vi "DC Offset.vi"() -> ()   [LabVIEW 2018]
uses:
  <vilib>/Analysis/baseanly.llb/Mean (DBL).vi
  <vilib>/express/express shared/transition.llb/Dynamic To Waveform Array.vi
  <vilib>/express/express signal manip/GetorSetDDTAttributes/Set DDT Attributes/SetT0.vi
  <vilib>/express/express shared/transition.llb/Waveform Array To Dynamic.vi
  <vilib>/express/express signal manip/GetorSetDDTAttributes/Set DDT Attributes/Set DDT Properties.xnode
  <vilib>/Analysis/NI_AALBase.lvlib
panel:
  in  "Filename":path=path "C:/Users/physics-svc-fulda/Desktop/LabVIEW Data/DC OFFset.lvm"
  out "Waveform Graph":dynamicdata(graph)
  out "Saving Data":bool
  in  "Enable":bool=TRUE
  out "DC D":dbl format="%0.6f"
  out "DC C":dbl format="%0.6f"
  out "DC B":dbl format="%0.6f"
  out "DC A":dbl format="%0.6f"
  in  "timeout (s)":dbl=10.0 format="%0.2f"
  in  "rate":dbl=1000.0
  in  "# of samples":i32=100
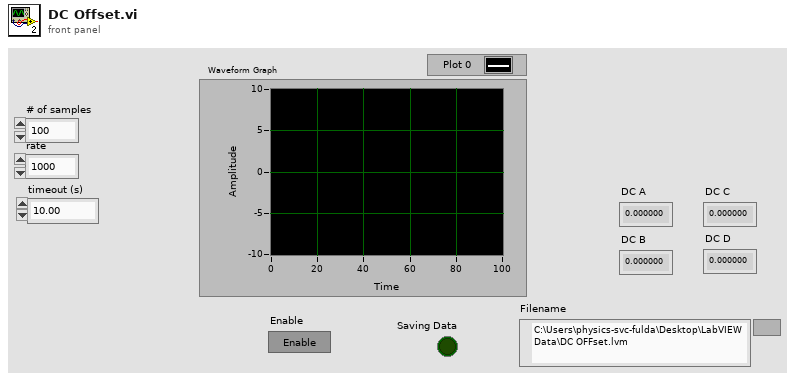
[diagram p1: front panel]
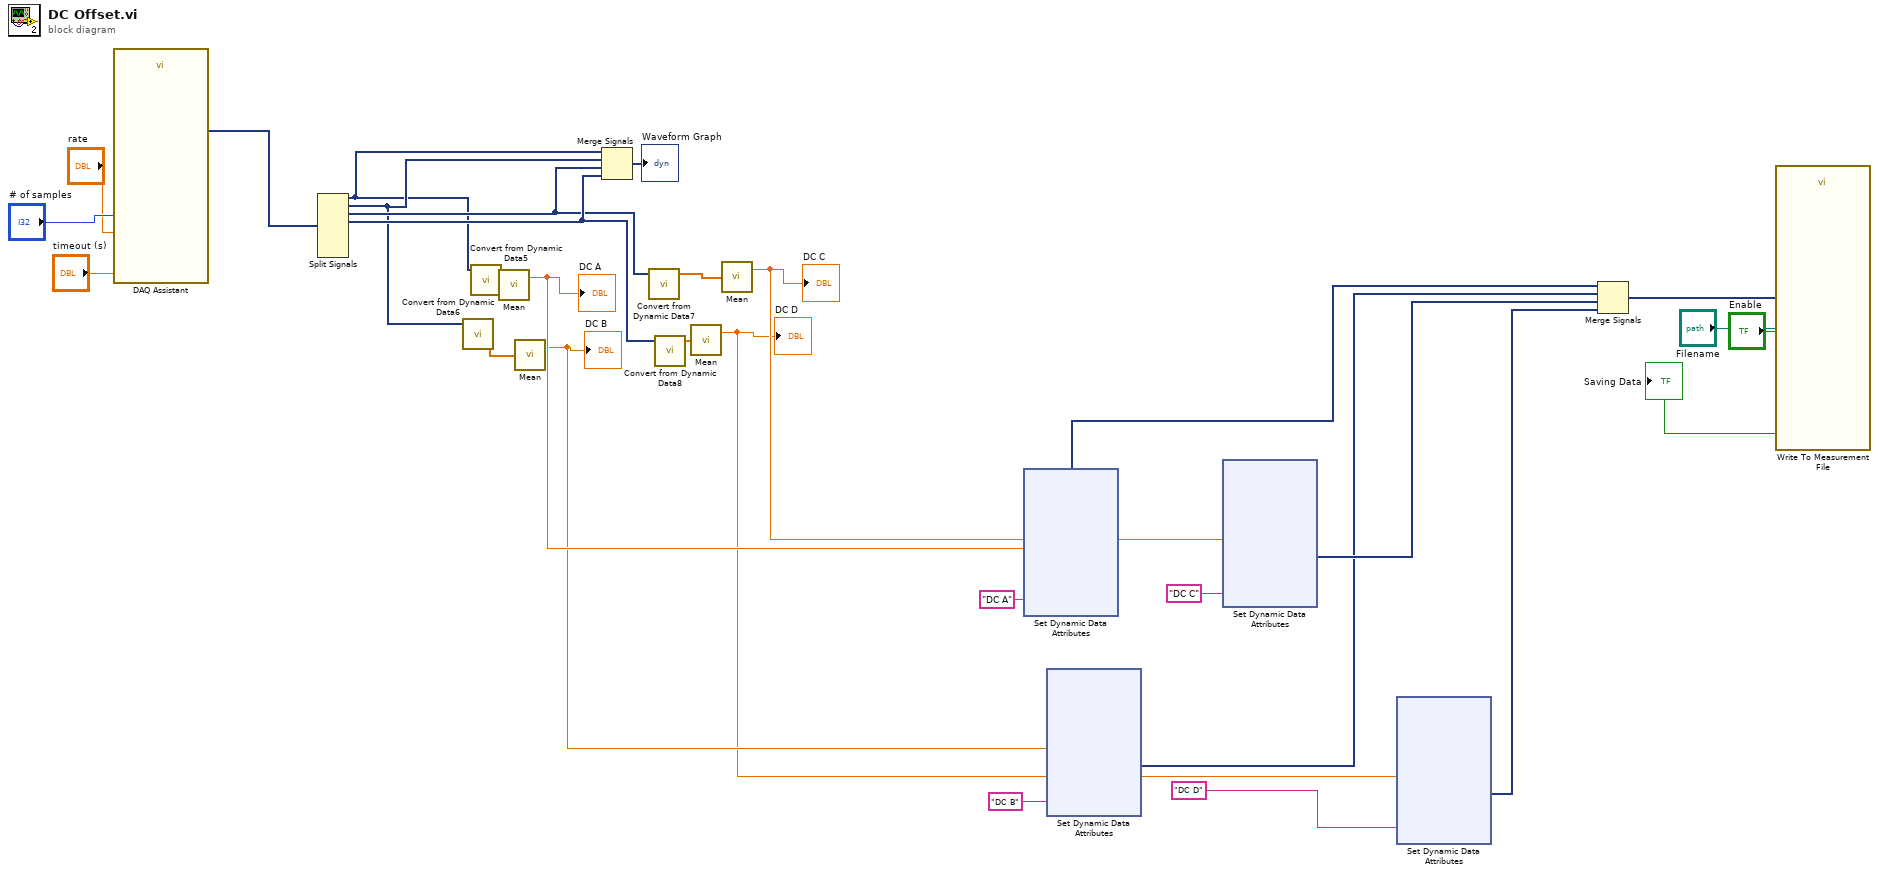
[diagram p0: block diagram]
diagram:
  n1 = call "DAQ Assistant"("rate"="rate", "number of samples"="# of samples", "timeout (s)"="timeout (s)") -> ("data"=w26:dynamicdata)  [unwired: 14 in, 2 out]
  n2 = Split Signals(w26) -> (w2:dynamicdata, w3:dynamicdata, w4:dynamicdata, w5:dynamicdata)  [unwired: 8 in, 4 out]
  n3 = call "Convert from Dynamic Data6"("Dynamic Data Type"=w3) -> ("Array"=w24:dbl[])  [unwired: 3 in]
  n4 = call "Convert from Dynamic Data5"("Dynamic Data Type"=w2) -> ("Array"=w25:dbl[])  [unwired: 3 in]
  n5 = call-poly <vilib>:"Mean.vi"("X"=w25) -> ("mean"=w18:dbl)  [unwired: 1 out]
  "DC A" <- w18
  n6 = call-poly <vilib>:"Mean.vi"("X"=w24) -> ("mean"=w17:dbl)  [unwired: 1 out]
  "DC B" <- w17
  n7 = Merge Signals(w2, w3, w4, w5) -> (→"Waveform Graph":dynamicdata)
  n8 = call "Convert from Dynamic Data7"("Dynamic Data Type"=w4) -> ("Array"=w23:dbl[])  [unwired: 3 in]
  n9 = call "Convert from Dynamic Data8"("Dynamic Data Type"=w5) -> ("Array"=w22:dbl[])  [unwired: 3 in]
  n10 = call-poly <vilib>:"Mean.vi"("X"=w22) -> ("mean"=w15:dbl)  [unwired: 1 out]
  "DC D" <- w15
  n11 = call-poly <vilib>:"Mean.vi"("X"=w23) -> ("mean"=w16:dbl)  [unwired: 1 out]
  "DC C" <- w16
  n12 = xnode "Set Dynamic Data Attributes"("Signals In"=w18, "Signal Name"="DC A") -> ("Signals Out"=w10:dynamicdata)  [unwired: 2 in, 1 out]
  n13 = xnode "Set Dynamic Data Attributes"("Signals In"=w17, "Signal Name"="DC B") -> ("Signals Out"=w8:dynamicdata)  [unwired: 2 in, 1 out]
  n14 = xnode "Set Dynamic Data Attributes"("Signals In"=w16, "Signal Name"="DC C") -> ("Signals Out"=w9:dynamicdata)  [unwired: 2 in, 1 out]
  n15 = xnode "Set Dynamic Data Attributes"("Signals In"=w15, "Signal Name"="DC D") -> ("Signals Out"=w7:dynamicdata)  [unwired: 2 in, 1 out]
  n16 = Merge Signals(w10, w8, w9, w7) -> (w21:dynamicdata)
  n17 = call "Write To Measurement File"("Signals"=w21, "Enable"="Enable", "Filename"="Filename") -> ("Saving Data"=→"Saving Data":bool)  [unwired: 14 in, 2 out]
